vi "Check Msg.vi"(9 "Msg":refnum<class "Msg.lvclass">, 10 "Msg Attributes":refnum<data-value>) -> (2 "Match":bool)   [LabVIEW 2020, in "jettl.lvlib"]
uses:
  jettl.lvlib
  Msg/Msg.lvclass
  Msg Input/Msg Input.lvclass
  Msg Output/Msg Output.lvclass
  Transport/Transport.lvclass
  Relation.ctl
  Teller.ctl
  Msg Attributes.ctl
  Msgs.ctl
  Unified Layer.ctl
  Actor Attributes.ctl
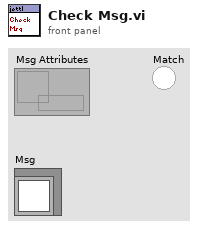
[diagram p1: front panel]
types:
  T1 = typedef "jettl.lvlib/Msg Attributes.ctl" = cluster{"Msg":refnum<class "Msg.lvclass">, "Msg Input":refnum<class "Msg Input.lvclass">, "Msg Output":refnum<class "Msg Output.lvclass">, "Teller":refnum<data-value>}
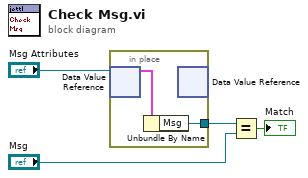
[diagram p0: block diagram]
diagram:
  n1 = in-place {
    in-place-border: [w5] -> w1
    n2 = in-place-dvr #1("Msg Attributes") -> (w6:T1)  [unwired: 1 out]
    n3 = Unbundle By Name(w6) -> ("Msg"=w5:refnum<class "Msg.lvclass">)
    n4 = in-place-dvr #1() -> ()  [unwired: 1 in, 2 out]
  }
  n5 = Equal?(x=w1, y="Msg") -> (x = y?=→"Match":bool)
